vi "FindLibraryParent.vi"(8 "error in":errorcluster, 11 "ProjectItem":refnum<vi>) -> (0 "error out":errorcluster, 3 "LibraryItem":refnum<vi>)   [LabVIEW 2017, in "NI_Variable.lvlib"]
uses:
  <vilib>/variable/NI_Variable.lvlib
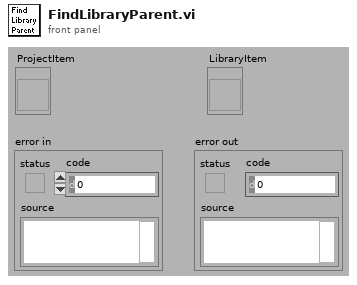
[diagram p1: front panel]
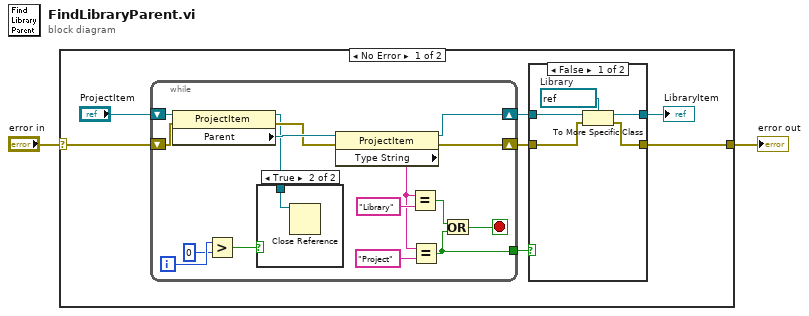
[diagram p0: block diagram]
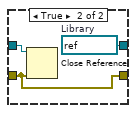
[diagram p2: hidden frame]
diagram:
  n1 = case shown="No Error" "error in" {
    selector: "error in" -> [w8 w35]
    tunnel: [w4 w35] -> w1
    frame No Error {
      n2 = while {
        shift-right: [w31] -> w7
        shift-left: "ProjectItem" -> [w33]
        shift-right: [w29] -> w5
        shift-left: w8 -> [w30]
        tunnel: [w23] -> w3
        i -> [w20]
        stop <- w24 stop-if-true
        n3 = property class="ProjectItem"(reference=w33, error in=w30) -> (reference out=w21:refnum<vi>, error out=w22:errorcluster, "Parent"=w32:refnum<vi>)
        n4 = Greater?(x=w20, y=0) -> (0:w18:bool)
        n5 = case shown="True" w18 {
          tunnel: w21 -> [_ w34]
          frame False {
          }
          frame True {
            n6 = Close Reference(reference=w34) -> ()  [unwired: 1 in, 1 out]
          }
        }
        n7 = property class="ProjectItem"(reference=w32, error in=w22) -> (reference out=w31:refnum<vi>, error out=w29:errorcluster, "Type String"=w27:string)
        n8 = Equal?(x=w27, y="Library") -> (x = y?=w25:bool)
        n9 = Equal?(x=w27, y="Project") -> (x = y?=w23:bool)
        n10 = Or(x=w25, y=w23) -> (x .or. y?=w24:bool)
      }
      n11 = case shown="False" w3 {
        tunnel: w7 -> [w14 w16]
        tunnel: [w12 w17] -> w6
        tunnel: w5 -> [w11 w15]
        tunnel: [w10 w15] -> w4
        frame False {
          w13 = refnum<vi> refnum  # Library
          n12 = To More Specific Class(target class=w13, reference=w14, error in=w11) -> (specific class reference=w12:refnum<vi>, error out=w10:errorcluster)
        }
        frame True {
          w17 = refnum<vi> refnum  # Library
          n13 = Close Reference(reference=w16, error in (no error)=w15) -> ()  [unwired: 1 out]
        }
      }
      "LibraryItem" <- w6
    }
    frame Error {
    }
  }
  "error out" <- w1
